vi "Gripper Status.vi"(8 "error in":errorcluster, 9 "Input":cluster{"Left":dbl, "Right":dbl}, 10 "Moving? (F)":bool, 11 "Action":T1) -> (0 "error out":errorcluster, 2 "Gripper SP":cluster{"Left":dbl, "Right":dbl}, 3 "Moving?":bool)   [LabVIEW 2017]
uses:
  Typedef/FGVAction.ctl
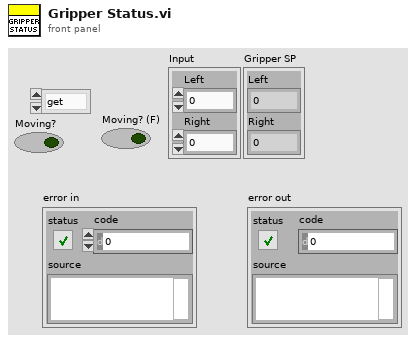
[diagram p1: front panel]
types:
  T1 = typedef "FGVAction.ctl" = enum16{"get", "set"}
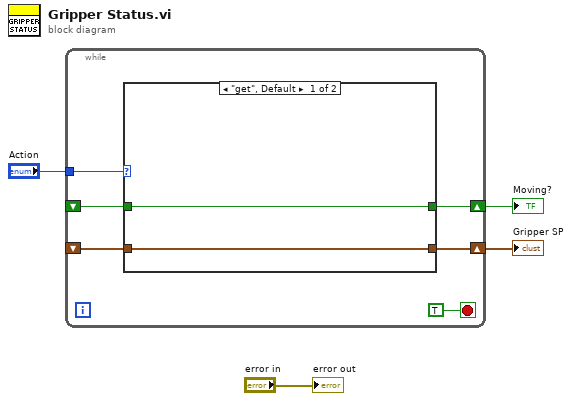
[diagram p0: block diagram]
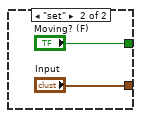
[diagram p2: hidden frame]
diagram:
  n1 = while {
    tunnel: "Action" -> [w10]
    shift-right: [w9] -> w2
    shift-left: _ -> [w8]
    shift-right: [w6] -> w1
    shift-left: _ -> [w5]
    stop <- TRUE stop-if-true
    n2 = case shown="\"get\", Default" w10 {
      tunnel: [w12 "Moving? (F)"] -> w9
      tunnel: w8 -> [w12 _]
      tunnel: [w11 "Input"] -> w6
      tunnel: w5 -> [w11 _]
      frame "get", Default {
      }
      frame "set" {
      }
    }
  }
  "Moving?" <- w2
  "Gripper SP" <- w1
  "error out" <- "error in"
